vi "SSL_Read.vi"(6 "timeout ms (5000)":i32=5000, 8 "error in (no error)":errorcluster, 10 "bytes to read":i32, 11 "SSL_Connection":T1) -> (0 "error out":errorcluster, 1 "timeout?":bool, 2 "data out":u8[](array[numeric]) format="%x", 3 "SSL_Connection":T1)   [LabVIEW 2018, in "AWS_IoT.lvlib"]
doc: "read num bytes from the specified ssl into the buffer\n\nDistributed under the MIT License\n\nCopyright (c) 2016 Indie-Energy\n\nPermission is hereby granted, free of charge, to any person obtaining a copy\nof this software and associated documentation files (the \"Software\"), to deal\nin the Software without restriction, including without limitation the rights\nto use, copy, modify, merge, publish, distribute, sublicense, and/or sell\ncopies of the Software, and to permit persons to whom the Software is\nfurnished to do so, subject to the following conditions:\n\nThe above copyright notice and this permission notice shall be included in all\ncopies or substantial portions of the Software.\n\nTHE SOFTWARE IS PROVIDED \"AS IS\", WITHOUT WARRANTY OF ANY KIND, EXPRESS OR\nIMPLIED, INCLUDING BUT NOT LIMITED TO THE WARRANTIES OF MERCHANTABILITY,\nFITNESS FOR A PARTICULAR PURPOSE AND NONINFRINGEMENT. IN NO EVENT SHALL THE\nAUTHORS OR COPYRIGHT HOLDERS BE LIABLE FOR ANY CLAIM, DAMAGES OR OTHER\nLIABILITY, WHETHER IN AN ACTION OF CONTRACT, TORT OR OTHERWISE, ARISING FROM,\nOUT OF OR IN CONNECTION WITH THE SOFTWARE OR THE USE OR OTHER DEALINGS IN THE\nSOFTWARE."
uses:
  AWS_IoT.lvlib
  Controls/SSL_Connection.ctl
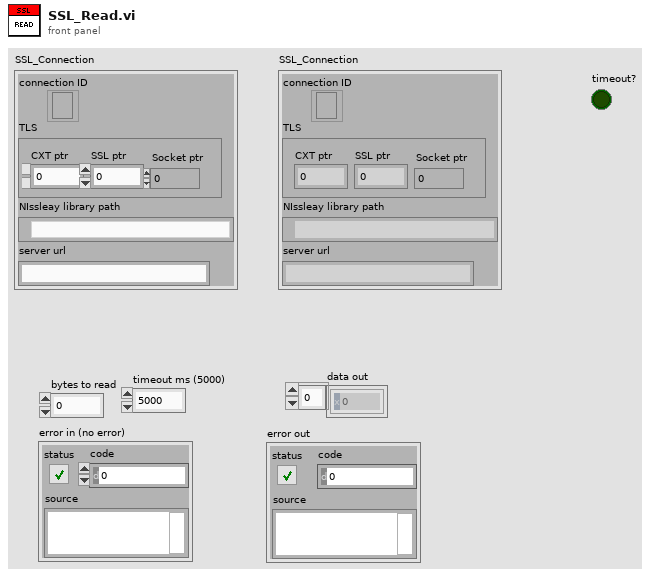
[diagram p1: front panel]
types:
  T1 = typedef "AWS_IoT.lvlib/SSL_Connection.ctl" = cluster{"connection ID":refnum<k5>, "TLS":cluster{"CXT ptr":i32, "SSL ptr":i32, "Socket ptr":i32}, "NIssleay library path":path, "server url":string}
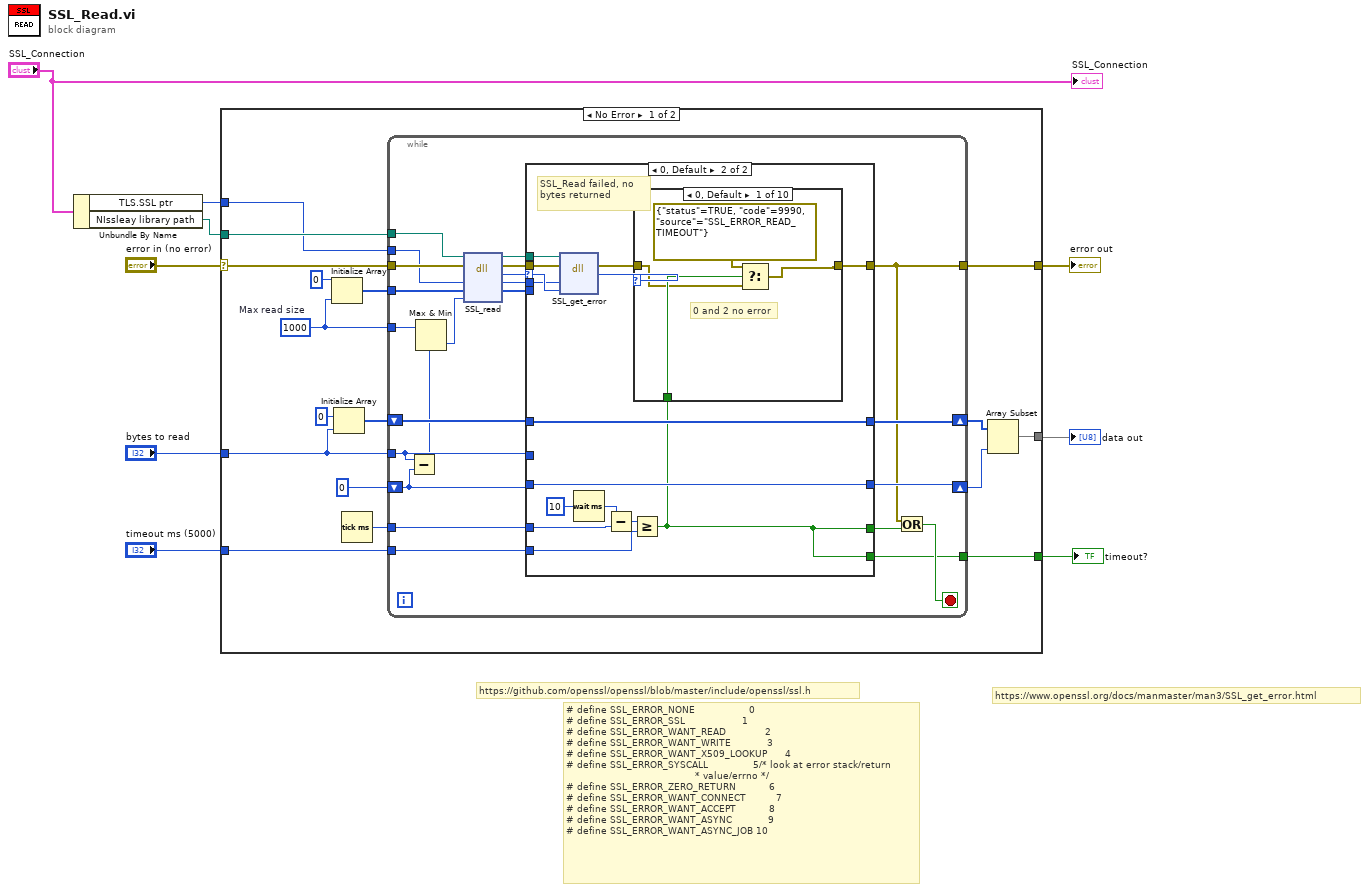
[diagram p0: block diagram]
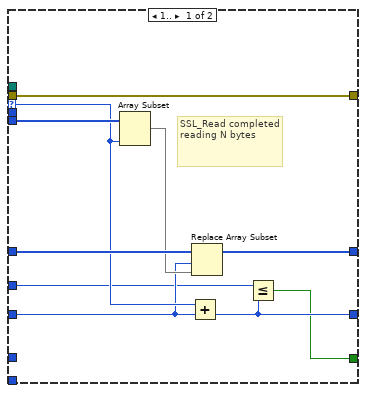
[diagram p2: hidden frame]
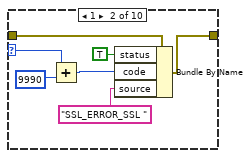
[diagram p3: hidden frame]
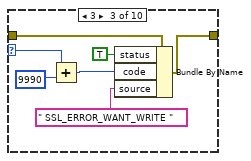
[diagram p4: hidden frame]
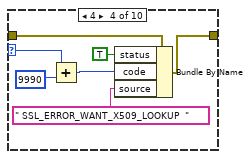
[diagram p5: hidden frame]
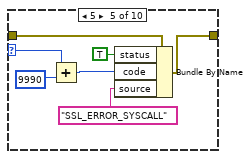
[diagram p6: hidden frame]
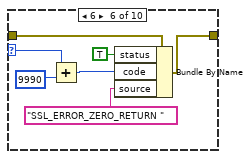
[diagram p7: hidden frame]
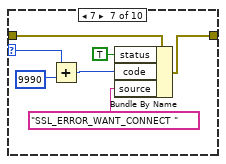
[diagram p8: hidden frame]
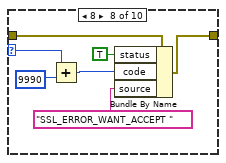
[diagram p9: hidden frame]
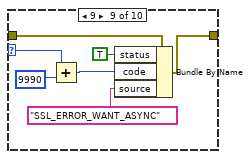
[diagram p10: hidden frame]
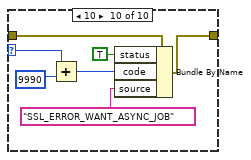
[diagram p11: hidden frame]
diagram:
  # "https://github.com/openssl/openssl/blob/master/include/openssl/ssl.h"
  # "https://www.openssl.org/docs/manmaster/man3/SSL_get_error.html"
  # "# define SSL_ERROR_NONE                  0\n# define SSL_ERROR_SSL                   1\n# define SSL_ERROR_WANT_READ             2\n# define SSL_ERROR_WANT_WRITE            3\n# define SSL_ERROR_WANT_X509_LOOKUP      4\n# define SSL_ERROR_SYSCALL               5/* look at error stack/return\n                                           * value/errno */\n# define SSL_ERROR_ZERO_RETURN           6\n# define SSL_ERROR_WANT_CONNECT          7\n# define SSL_ERROR_WANT_ACCEPT           8\n# define SSL_ERROR_WANT_ASYNC            9\n# define SSL_ERROR_WANT_ASYNC_JOB 10"
  n1 = Unbundle By Name("SSL_Connection") -> ("TLS.SSL ptr"=w6:i32, "NIssleay library path"=w8:path)
  n2 = case shown="No Error" "error in (no error)" {
    selector: "error in (no error)" -> [w25 w142]
    tunnel: w8 -> [w26 _]
    tunnel: w6 -> [w24 _]
    tunnel: "bytes to read" -> [w19 _]
    tunnel: [w14 _] -> w4
    tunnel: [w13 w142] -> w3
    tunnel: "timeout ms (5000)" -> [w11 _]
    tunnel: [w10 _] -> w1
    frame No Error {
      w21 = 1000  # Max read size
      n3 = Initialize Array(u8 0 ("element"), w21) -> (w22:u8[])
      n4 = Initialize Array(u8 0 ("element"), w19) -> (w18:u8[])
      n5 = Tick Count (ms)() -> (millisecond timer value=w12:u32)
      n6 = while {
        tunnel: w26 -> [w49]
        tunnel: w25 -> [w48]
        tunnel: w24 -> [w47]
        tunnel: w19 -> [w38]
        tunnel: w22 -> [w42]
        tunnel: w21 -> [w41]
        shift-right: [w39] -> w16
        shift-left: w18 -> [w40]
        shift-right: [w33] -> w15
        shift-left: 0 -> [w34]
        tunnel: [w31] -> w13
        tunnel: w12 -> [w29]
        tunnel: w11 -> [w28]
        tunnel: [w27] -> w10
        stop <- w32 stop-if-true
        n7 = Subtract(x=w38, y=w34) -> (x-y=w37:i32)
        n8 = Max & Min(x=w41, y=w37) -> (min(x,y)=w43:i32)  [unwired: 1 out]
        n9 = dll-call lib="NIssleay32.*" fn="SSL_read"(path in=w49, error in=w48, "SSL"=w47, "stringBuf"=w42, "stringLen"=w43) -> (path out=w44:path, error out=w45:errorcluster, "noOfBytes"=w46:i32, "SSL"=w35:i32, "stringBuf"=w36:u8[])  [unwired: 2 in]
        n10 = case shown="0, Default" w46 {
          selector: w46 -> [w54 w71]
          tunnel: w44 -> [_ w69]
          tunnel: w45 -> [w59 w72]
          tunnel: [w59 w61] -> w31
          tunnel: [w50 w60] -> w30
          tunnel: w36 -> [w58 _]
          tunnel: w40 -> [w57 w74]
          tunnel: [w56 w74] -> w39
          tunnel: w34 -> [w53 w73]
          tunnel: [w52 w73] -> w33
          tunnel: w38 -> [w51 _]
          tunnel: w35 -> [_ w70]
          tunnel: w29 -> [_ w65]
          tunnel: w28 -> [_ w64]
          tunnel: [_ w60] -> w27
          frame 1.. {
            # "SSL_Read completed reading N bytes"
            n11 = Array Subset(array=w58, length=w54) -> (w55:u8[])  [unwired: 1 in]
            n12 = Add(x=w54, y=w53) -> (x+y=w52:i32)
            n13 = Replace Array Subset(array=w57, new element=w55, index=w53) -> (w56:u8[])
            n14 = Less Or Equal?(x=w51, y=w52) -> (x <= y?=w50:bool)
          }
          frame 0, Default {
            # "SSL_Read failed, no bytes returned"
            n15 = dll-call lib="NIssleay32.*" fn="SSL_get_error"(path in=w69, error in=w72, "SSL"=w70, "retCode"=w71) -> (error out=w62:errorcluster, "return type"=w63:i32)  [unwired: 3 in, 1 out]
            n16 = Wait (ms)(milliseconds to wait=u32 10) -> (millisecond timer value=w68:u32)
            n17 = Subtract(x=w68, y=w65) -> (x-y=w66:u32)
            n18 = Greater Or Equal?(x=w66, y=w64) -> (x >= y?=w60:bool)
            n19 = case shown="0, Default" w63 {
              selector: w63 -> [_ w82 w89 w96 w103 w110 w117 w124 w131 w138]
              tunnel: w62 -> [w77 w85 w92 w99 w106 w113 w120 w127 w134 w141]
              tunnel: [w76 w84 w91 w98 w105 w112 w119 w126 w133 w140] -> w61
              tunnel: w60 -> [w78 _ _ _ _ _ _ _ _ _]
              frame 0, Default {
                # "0 and 2 no error"
                n20 = Select(t=errorcluster {"status"=TRUE, "code"=9990, "source"="SSL_ERROR_READ_TIMEOUT"}, s=w78, f=w77) -> (s? t:f=w76:errorcluster)
              }
              frame 1 {
                n21 = Add(x=w82, y=9990) -> (x+y=w80:i32)
                n22 = Bundle By Name(cluster=w85, "status"=TRUE, "code"=w80, "source"="SSL_ERROR_SSL ") -> (w84:errorcluster)
              }
              frame 3 {
                n23 = Add(x=w89, y=9990) -> (x+y=w87:i32)
                n24 = Bundle By Name(cluster=w92, "status"=TRUE, "code"=w87, "source"=" SSL_ERROR_WANT_WRITE ") -> (w91:errorcluster)
              }
              frame 4 {
                n25 = Add(x=w96, y=9990) -> (x+y=w94:i32)
                n26 = Bundle By Name(cluster=w99, "status"=TRUE, "code"=w94, "source"=" SSL_ERROR_WANT_X509_LOOKUP  ") -> (w98:errorcluster)
              }
              frame 5 {
                n27 = Add(x=w103, y=9990) -> (x+y=w101:i32)
                n28 = Bundle By Name(cluster=w106, "status"=TRUE, "code"=w101, "source"="SSL_ERROR_SYSCALL") -> (w105:errorcluster)
              }
              frame 6 {
                n29 = Add(x=w110, y=9990) -> (x+y=w108:i32)
                n30 = Bundle By Name(cluster=w113, "status"=TRUE, "code"=w108, "source"="SSL_ERROR_ZERO_RETURN ") -> (w112:errorcluster)
              }
              frame 7 {
                n31 = Add(x=w117, y=9990) -> (x+y=w115:i32)
                n32 = Bundle By Name(cluster=w120, "status"=TRUE, "code"=w115, "source"="SSL_ERROR_WANT_CONNECT ") -> (w119:errorcluster)
              }
              frame 8 {
                n33 = Add(x=w124, y=9990) -> (x+y=w122:i32)
                n34 = Bundle By Name(cluster=w127, "status"=TRUE, "code"=w122, "source"="SSL_ERROR_WANT_ACCEPT ") -> (w126:errorcluster)
              }
              frame 9 {
                n35 = Add(x=w131, y=9990) -> (x+y=w129:i32)
                n36 = Bundle By Name(cluster=w134, "status"=TRUE, "code"=w129, "source"="SSL_ERROR_WANT_ASYNC") -> (w133:errorcluster)
              }
              frame 10 {
                n37 = Add(x=w138, y=9990) -> (x+y=w136:i32)
                n38 = Bundle By Name(cluster=w141, "status"=TRUE, "code"=w136, "source"="SSL_ERROR_WANT_ASYNC_JOB") -> (w140:errorcluster)
              }
            }
          }
        }
        n39 = Or(x=w31, y=w30) -> (x .or. y?=w32:bool)
      }
      n40 = Array Subset(array=w16, length=w15) -> (w14:u8[])  [unwired: 1 in]
    }
    frame Error {
    }
  }
  "data out" <- w4
  "error out" <- w3
  "timeout?" <- w1
  "SSL_Connection" <- "SSL_Connection"
